vi "全局变量.vi"() -> ()   [LabVIEW 2015]
panel:
  out "当前状态：":string
  out "时刻":T1={"点时间"=timestamp(3595558893.17812 s since 1904-01-01), "行时间"=timestamp(3595558891.757594 s since 1904-01-01), "层时间"=timestamp(3595558833.124629 s since 1904-01-01)}
  in  "打印设置":T2={"f_objecitve(mm)"=1.8, "f_tubelens(mm)"=200.0, "f_scanlens(mm)"=50.0, "模型高/um"=2.0, "XY速度(um/s) "=0.0, "比例因子(V/°)"=1.0}
  in  "I/O 设置":T3={"matlab函数目录"=path "C:/Users/eason/Documents/GitHub/TPP-3D-printer/Matlab", "读取点阵文件"=path "C:/Users/eason/Documents/GitHub/TPP-3D-printer/Matlab/grating.txt", "DO通道：shutter控制"="Dev1/port1/line0", "AO通道：X前Y后"="Dev1/ao0:1", "Z轴驱动序列号"="27002049"}
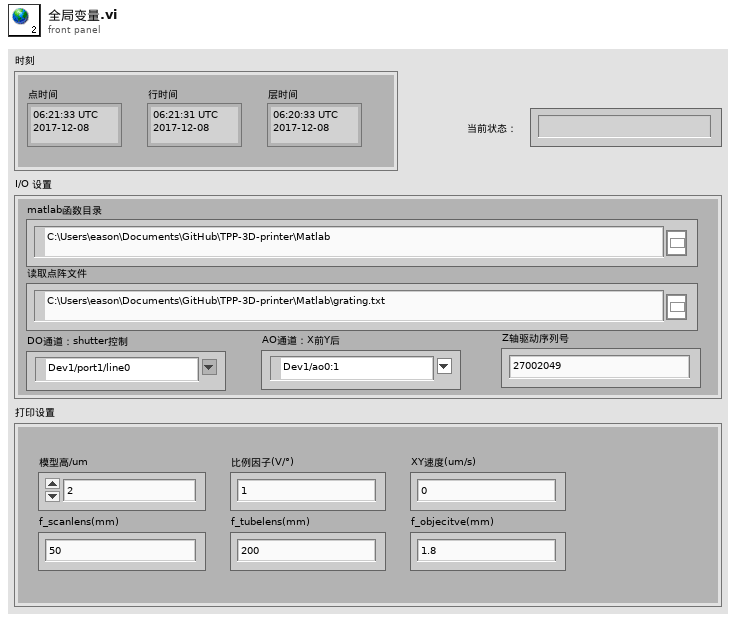
[diagram p1: front panel]
types:
  T1 = cluster{"点时间":timestamp, "行时间":timestamp, "层时间":timestamp}
  T2 = cluster{"f_objecitve(mm)":dbl, "f_tubelens(mm)":dbl, "f_scanlens(mm)":dbl, "模型高/um":dbl, "XY速度(um/s) ":dbl, "比例因子(V/°)":dbl}
  T3 = cluster{"matlab函数目录":path, "读取点阵文件":path, "DO通道：shutter控制":tag, "AO通道：X前Y后":tag, "Z轴驱动序列号":string}
diagram:
